vi "Initialize.vi"() -> (3 "Weights":cluster{"thetas":dbl[], "offset":dbl})   [LabVIEW 2014]
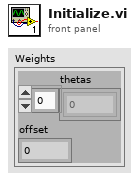
[diagram p1: front panel]
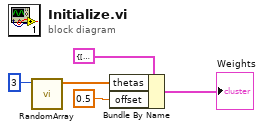
[diagram p0: block diagram]
diagram:
  n1 = call "RandomArray.vi"("Numeric"=3) -> ("Array"=w3:dbl[])  [unwired: 10 in]
  n2 = Bundle By Name(cluster=cluster{"thetas":dbl[], "offset":dbl} {"thetas"=[], "offset"=0.0} ("Weights"), "thetas"=w3, "offset"=0.5) -> (→"Weights":cluster{"thetas":dbl[], "offset":dbl})
